vi "ToUint16.vi"(1 "index":i32, 2 "array":u8[](array[numeric])) -> (0 "sp float":u16)   [LabVIEW 2009]
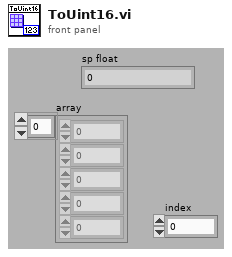
[diagram p1: front panel]
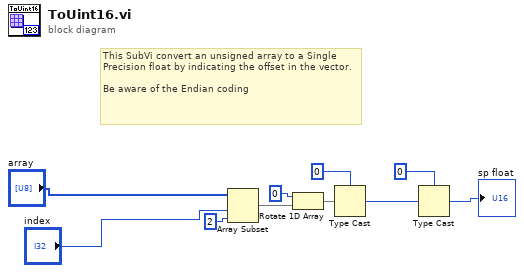
[diagram p0: block diagram]
diagram:
  # "This SubVi convert an unsigned array to a Single Precision float by indicating the offset in the vector.\n\nBe aware of the Endian coding"
  n1 = Array Subset(array="array", index="index", length=2) -> (w6:u8[])
  n2 = Rotate 1D Array(1:w6, 2:0 ("n")) -> (0:w4:u8[])
  n3 = Type Cast(type=u32 0 ("length"), x=w4) -> (*(type *) &x=w1:u32)
  n4 = Type Cast(type=u16 0 ("sp float"), x=w1) -> (*(type *) &x=→"sp float":u16)
